vi "parse.vi"(5 "ts least":timestamp, 6 "ts great":timestamp, 7 "iterative":i32, 9 "file path":path, 10 "Column Name":string) -> (0 "ts least":timestamp, 1 "ts great":timestamp, 2 "Array out":string[][](array[string]))   [LabVIEW 2017]
uses:
  <vilib>/Utility/file.llb/Read Delimited Spreadsheet (string).vi
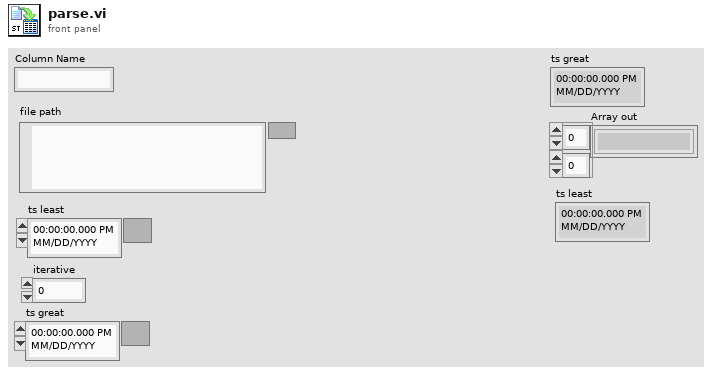
[diagram p1: front panel]
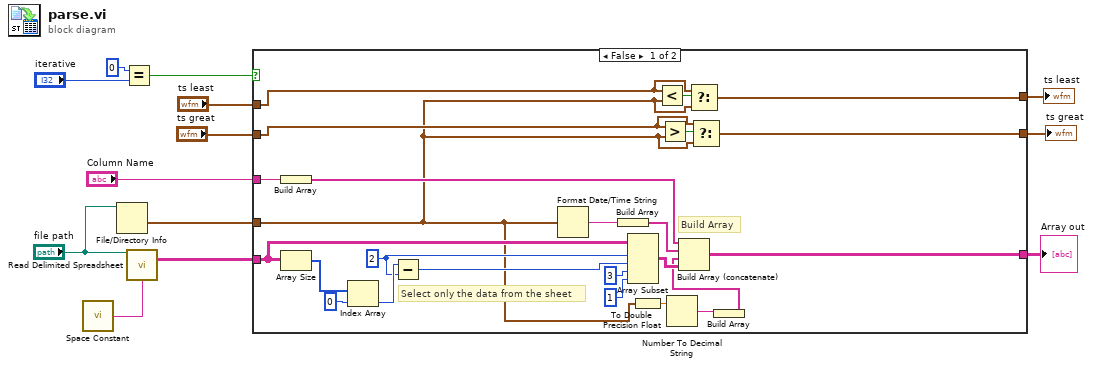
[diagram p0: block diagram]
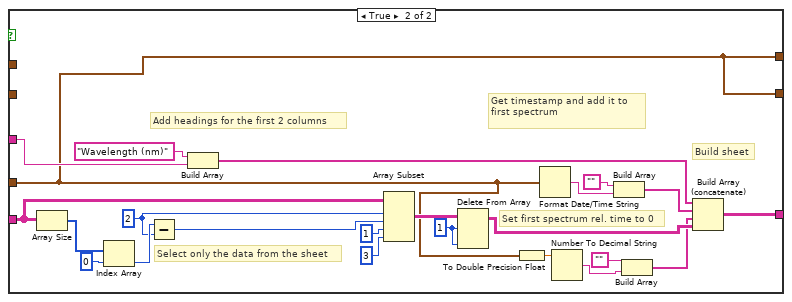
[diagram p2: hidden frame]
diagram:
  n1 = call <vilib>:"Space Constant.vi"() -> ("String"=w8:string)
  n2 = File/Directory Info(path="file path") -> (last mod=w6:timestamp)  [unwired: 1 in, 6 out]
  n3 = Equal?(x=0, y="iterative") -> (x = y?=w13:bool)
  n4 = call-poly <vilib>:"Read Delimited Spreadsheet.vi"("file path (dialog if empty)"="file path", "delimiter (\\t)"=w8) -> ("all rows"=w7:string[][])  [unwired: 8 in, 5 out]
  n5 = case shown="False" w13 {
    tunnel: w7 -> [w25 w50]
    tunnel: [w34 w51] -> w4
    tunnel: "Column Name" -> [w33 w52]
    tunnel: "ts least" -> [w23 _]
    tunnel: [w22 w38] -> w9
    tunnel: w6 -> [w14 w38]
    tunnel: "ts great" -> [w15 _]
    tunnel: [w17 w38] -> w1
    frame False {
      w26 = 2
      # "Build Array"
      # "Select only the data from the sheet"
      n6 = Build Array(w33) -> (w37:string[])
      n7 = Array Size(array=w25) -> (size(s)=w30:i32[])
      n8 = Index Array(array=w30, index=0) -> (element=w28:i32)
      n9 = Subtract(x=w28, y=w26) -> (x-y=w27:i32)
      n10 = Format Date/Time String(seconds (now)=w14) -> (date/time string=w36:string)  [unwired: 2 in]
      n11 = Build Array(w36) -> (w35:string[])
      n12 = Array Subset(array=w25, index (row)=w26, length (row)=w27, index (col)=3, length (col)=1) -> (w21:string[][])
      n13 = To Double Precision Float(number=w14) -> (double precision float=w19:dbl)
      n14 = Less?(x=w23, y=w14) -> (x < y?=w24:bool)
      n15 = Greater?(x=w15, y=w14) -> (0:w16:bool)
      n16 = Number To Decimal String(number=w19) -> (decimal integer string=w18:string)  [unwired: 1 in]
      n17 = Select(t=w23, s=w24, f=w14) -> (s? t:f=w22:timestamp)
      n18 = Select(t=w15, s=w16, f=w14) -> (s? t:f=w17:timestamp)
      n19 = Build Array(w18) -> (w20:string[])
      n20 = Build Array (concatenate)(w37, w35, w20, w21) -> (w34:string[][])
    }
    frame True {
      w59 = 1
      w45 = 2
      # "Build sheet"
      # "Set first spectrum rel. time to 0"
      # "Get timestamp and add it to first spectrum"
      # "Add headings for the first 2 columns"
      # "Select only the data from the sheet"
      n21 = Array Size(array=w50) -> (size(s)=w49:i32[])
      n22 = Index Array(array=w49, index=0) -> (element=w47:i32)
      n23 = Subtract(x=w47, y=w45) -> (x-y=w46:i32)
      n24 = Build Array("Wavelength (nm)", w52) -> (w56:string[])
      n25 = Array Subset(array=w50, index (row)=w45, length (row)=w46, index (col)=1, length (col)=3) -> (w60:string[][])
      n26 = Delete From Array(array=w60, length=w59, index (col)=w59) -> (array with subset deleted=w43:string[][])  [unwired: 1 in, 1 out]
      n27 = To Double Precision Float(number=w38) -> (double precision float=w42:dbl)
      n28 = Format Date/Time String(seconds (now)=w38) -> (date/time string=w54:string)  [unwired: 2 in]
      n29 = Number To Decimal String(number=w42) -> (decimal integer string=w40:string)  [unwired: 1 in]
      n30 = Build Array("", w54) -> (w53:string[])
      n31 = Build Array("", w40) -> (w39:string[])
      n32 = Build Array (concatenate)(w56, w53, w39, w43) -> (w51:string[][])
    }
  }
  "ts least" <- w9
  "Array out" <- w4
  "ts great" <- w1
